vi "Signal Out Single Point Cyclic.vi"() -> ()   [LabVIEW 2025]
uses:
  <vilib>/xnet/xnet.llb/XNET Create Session (Signal Output Single-point).vi
  <vilib>/xnet/xnet.llb/XNET Write (Signal Single-point).vi
panel:
  in  "Repetitions":u16(knob) scale=0.0..65535.0
  in  "signal list":refnum<k21>[](array[refnum])
  in  "Wait":u32=1000
  in  "stop":bool
  in  "interface":refnum<k21>="CAN1"
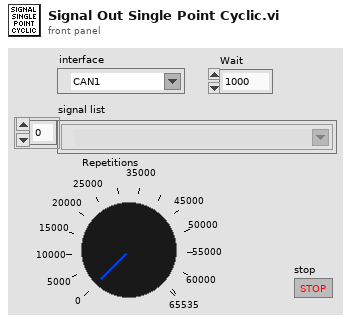
[diagram p1: front panel]
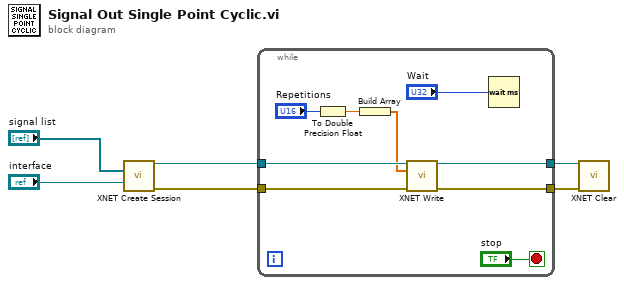
[diagram p0: block diagram]
diagram:
  n1 = call-poly <vilib>:"XNET Create Session.vi"("signal list"="signal list", "interface"="interface") -> ("session out"=w5:refnum<k21>, "error out"=w6:errorcluster)  [unwired: 12 in]
  n2 = while {
    tunnel: w6 -> [w14]
    tunnel: w5 -> [w15]
    tunnel: [w13] -> w3
    tunnel: [w12] -> w2
    stop <- "stop" stop-if-true
    n3 = To Double Precision Float(number="Repetitions") -> (double precision float=w7:dbl)
    n4 = Build Array(w7) -> (w8:dbl[])
    n5 = call-poly <vilib>:"XNET Write.vi"("session in"=w15, "data"=w8, "error in (no error)"=w14) -> ("session out"=w12:refnum<k21>, "error out"=w13:errorcluster)  [unwired: 11 in]
    n6 = Wait (ms)(milliseconds to wait="Wait") -> ()  [unwired: 1 out]
  }
  n7 = call <vilib>:"XNET Clear.vi"("session in"=w2, "error in (no error)"=w3) -> ()  [unwired: 13 in, 1 out]
